vi "UsrProfiles-Update last used profile ind.vi"(8 "error in":errorcluster) -> (0 "error out":errorcluster)   [LabVIEW 2013]
uses:
  Typedefs/Save-Load enum.ctl
  Globals/gl_UsrProfiles globals.vi
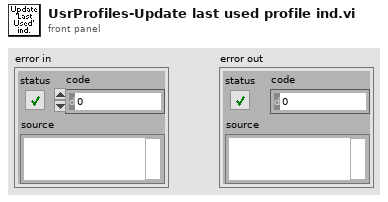
[diagram p1: front panel]
types:
  T1 = typedef "Save-Load enum.ctl" = enum16{"Save to file", "Load from file", "Compare from file"}
  T2 = typedef "User login window refs.ctl" = cluster{"User profiles window ref":refnum<k9>, "Users listbox":refnum<vi>, "Profiles listbox":refnum<vi>, "Last used":refnum<vi>}
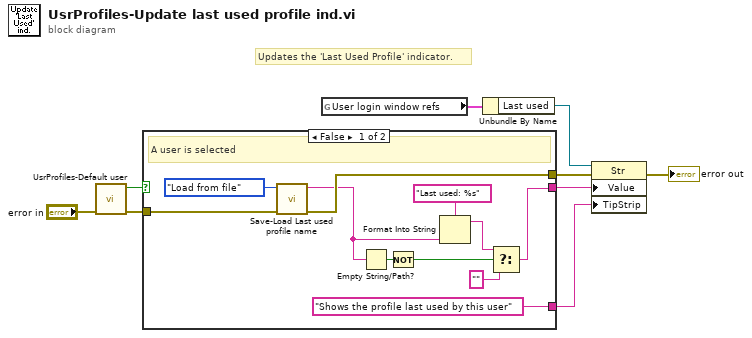
[diagram p0: block diagram]
diagram:
  # "Updates the 'Last Used Profile' indicator."
  n1 = call "UsrProfiles-Default user.vi"("error in (no error)"="error in") -> ("error out"=w4:errorcluster, "Default user selected"=w2:bool)  [unwired: 8 in, 1 out]
  n2 = case shown="False" w2 {
    tunnel: [w19 w21] -> w6
    tunnel: [w16 _] -> w5
    tunnel: w4 -> [w11 w21]
    tunnel: ["Shows the profile last used by this user" ("Tip Strip") _] -> w1
    frame False {
      # "A user is selected"
      n3 = call "Save-Load Last used profile name.vi"("error in"=w11, "Function"=Save-Load_enum."Load from file") -> ("error out"=w19:errorcluster, "Last used profile for selected user"=w13:string)  [unwired: 7 in, 1 out]
      n4 = Empty String/Path?(string/path=w13) -> (empty?=w18:bool)
      n5 = Not(x=w18) -> (.not. x?=w17:bool)
      n6 = Format Into String(format string="Last used: %s", w13) -> (resulting string=w12:string)  [unwired: 2 in, 1 out]
      n7 = Select(t=w12, s=w17, f="") -> (s? t:f=w16:string)
    }
    frame True {
      # "The Default User is selected."
    }
  }
  n8 = global read "gl_UsrProfiles globals.vi" "User login window refs"() -> (w8:T2)
  n9 = Unbundle By Name(w8) -> ("Last used"=w9:refnum<vi>)
  n10 = property on="Property Node" class="Str"(reference=w9, error in=w6, "Value"=w5, "TipStrip"=w1) -> (error out=→"error out":errorcluster)  [unwired: 1 out]
